vi "replace_ego_pose_legacy.vi"(4 "error in":errorcluster, 5 "Ego pose":T2={"angular velocity"=[0.0, 0.0, 0.0], "velocity"=[0.0, 0.0, 0.0], "steering_direction"=0.0, "position"=[0.0, 0.0, 0.0], "orientation YPR"={"yaw"=0.001, "pitch"=0.0, "roll"=0.0}} {"orientation YPR"."yaw" min=0.0 step=0.1 format="%#_5f"; "steering_direction" format="%#_13g"}, 6 "Frames":T1(array[cluster]), 7 "Frame number":i32) -> (0 "error out":errorcluster, 3 "Frame":string)   [LabVIEW 2019, in "Lib_Simx.lvlib"]
doc: "Replace the pose for the ego vehicle on a specific frame and outputs the JSON corresponding to the frame with the new settings."
uses:
  Lib_Simx.lvlib
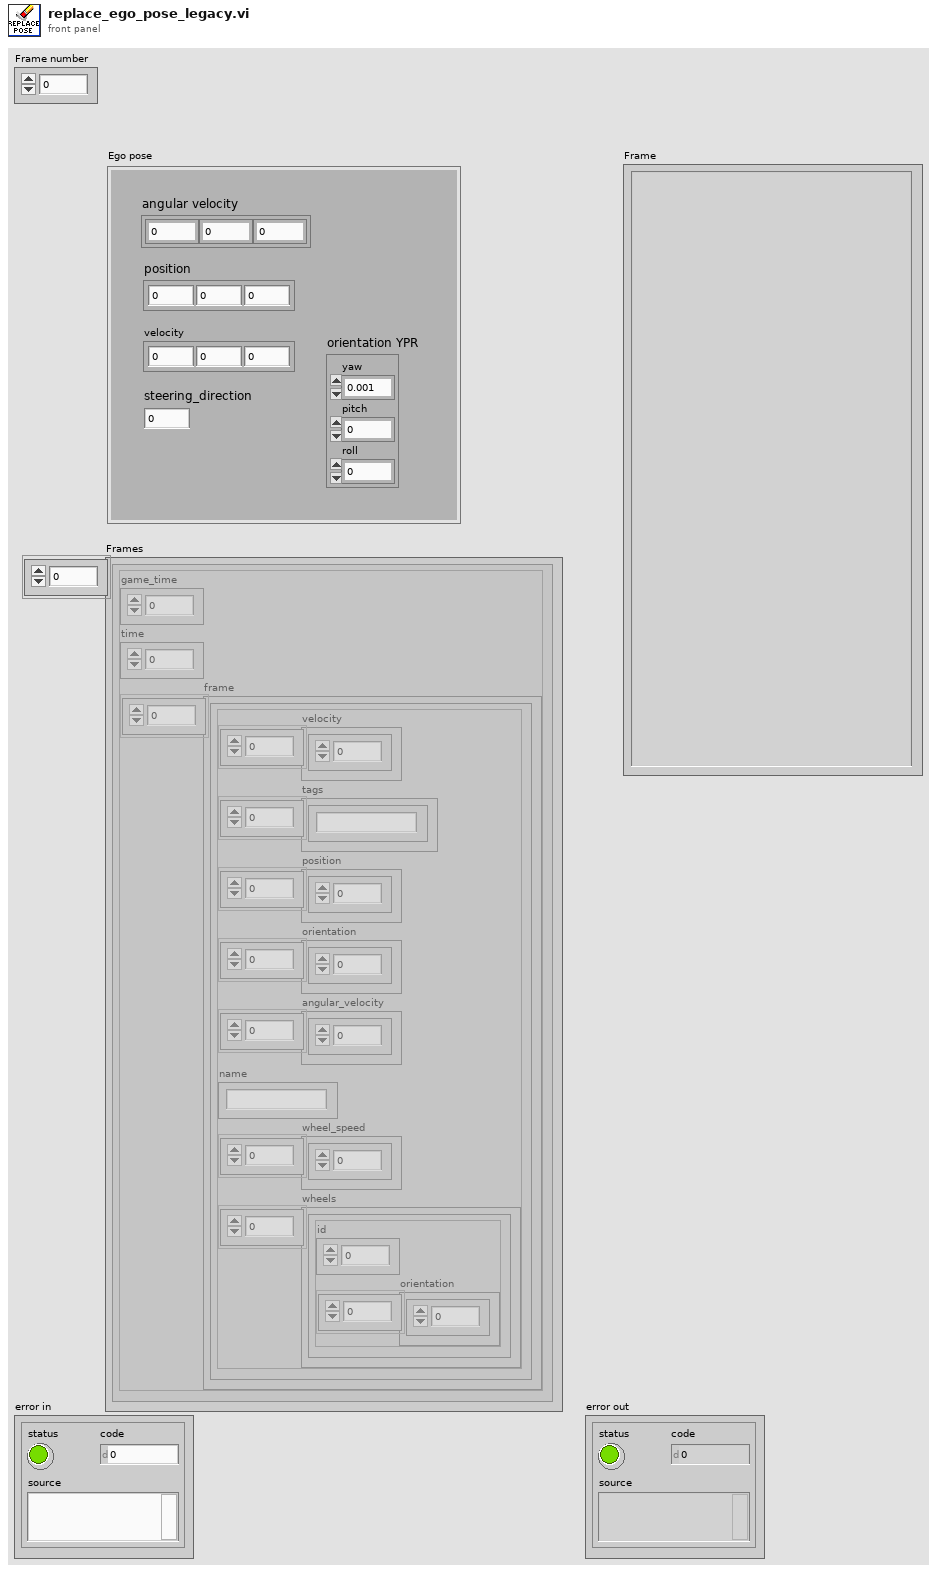
[diagram p1: front panel]
types:
  T1 = cluster{"game_time":dbl, "time":dbl, "frame":cluster{"velocity":dbl[], "tags":string[], "position":dbl[], "orientation":dbl[], "angular_velocity":dbl[], "name":string, "wheel_speed":dbl[], "wheels":cluster{"id":i32, "orientation":dbl[]}[]}[]}[]
  T2 = cluster{"angular velocity":dbl[], "velocity":dbl[], "steering_direction":dbl, "position":dbl[], "orientation YPR":cluster{"yaw":dbl, "pitch":dbl, "roll":dbl}}
  T3 = cluster{"game_time":dbl, "time":dbl, "frame":cluster{"velocity":dbl[], "tags":string[], "position":dbl[], "orientation":dbl[], "angular_velocity":dbl[], "name":string, "wheel_speed":dbl[], "wheels":cluster{"id":i32, "orientation":dbl[]}[]}[]}
  T4 = cluster{"velocity":dbl[], "tags":string[], "position":dbl[], "orientation":dbl[], "angular_velocity":dbl[], "name":string, "wheel_speed":dbl[], "wheels":cluster{"id":i32, "orientation":dbl[]}[]}[]
  T5 = cluster{"velocity":dbl[], "tags":string[], "position":dbl[], "orientation":dbl[], "angular_velocity":dbl[], "name":string, "wheel_speed":dbl[], "wheels":cluster{"id":i32, "orientation":dbl[]}[]}
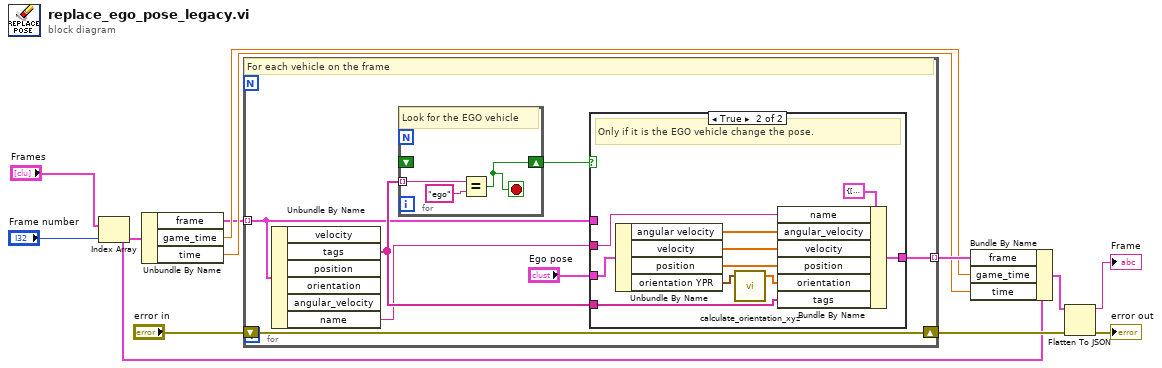
[diagram p0: block diagram]
diagram:
  n1 = Index Array(array="Frames", index="Frame number") -> (element=w2:T3)
  n2 = Unbundle By Name(w2) -> ("frame"=w6:T4, "game_time"=w7:dbl, "time"=w8:dbl)
  n3 = for {
    tunnel: w6 -> [w16] mode=indexing
    tunnel: [w15] -> w9 mode=indexing
    shift-right: [w14] -> w12
    shift-left: "error in" -> [w14]
    # "For each vehicle on the frame"
    n4 = Unbundle By Name(w16) -> ("tags"=w19:string[], "name"=w17:string)  [unwired: 4 out]
    n5 = for {
      tunnel: w19 -> [w33] mode=indexing
      shift-right: [w31] -> w18
      shift-left: _ -> [_]
      stop <- w31 stop-if-true
      # "Look for the EGO vehicle"
      n6 = Equal?(x=w33, y="ego") -> (x = y?=w31:bool)
    }
    n7 = case shown="True" w18 {
      tunnel: w19 -> [_ w25]
      tunnel: w17 -> [_ w30]
      tunnel: w16 -> [w20 _]
      tunnel: [w20 w24] -> w15
      tunnel: "Ego pose" -> [_ w29]
      frame False {
        # "Send the values without change for other vehicles"
      }
      frame True {
        # "Only if it is the EGO vehicle change the pose."
        n8 = Unbundle By Name(w29) -> ("angular velocity"=w28:dbl[], "velocity"=w27:dbl[], "position"=w26:dbl[], "orientation YPR"=w23:cluster{"yaw":dbl, "pitch":dbl, "roll":dbl})
        n9 = call "calculate_orientation_xyz.vi"("orientation YPR"=w23) -> ("pose"=w22:dbl[])  [unwired: 4 in]
        n10 = Bundle By Name(cluster=T5 {"velocity"=[], "tags"=[], "position"=[], "orientation"=[], "angular_velocity"=[], "name"="", "wheel_speed"=[], "wheels"=[]}, "name"=w30, "angular_velocity"=w28, "velocity"=w27, "position"=w26, "orientation"=w22, "tags"=w25) -> (w24:T5)
      }
    }
  }
  n11 = Bundle By Name(cluster=w2, "frame"=w9, "game_time"=w7, "time"=w8) -> (w10:T3)
  n12 = Flatten To JSON(anything=w10, error in (no error)=w12) -> (JSON string=→"Frame":string, 11:→"error out":errorcluster)  [unwired: 1 in]
